vi "TTB Convert.vi"(0 "time of 1st frame, sec since 1/1/04":dbl format="%.2f", 2 "First element of TTB values":u32, 3 "Current element of TTB values":u32) -> (5 "TTB Cluster Out":cluster{i32, u16, i16, i16})   [LabVIEW 2011]
doc: "Time Table Conversion VI.\n\n This VI converts a single element of the time table array by subtracting the first element from the current element. The number found is how many milliseconds have passed since the first frame grab. This information is stored in the TTB cluster in two ways: First, the number of seconds since 1970 is saved in the first slot of the cluster, then the number of milliseconds (three decimal places recorded) is saved in the second slot. The remaining two slots of the cluster are filled with zeros, as they are useless placeholders to make our TTB compliant with the C++ version.\n The VI divides the # of millisecs since the first frame by 1000 to achieve two goals: First, the quotient is added to the # of seconds to get the true # of seconds since the first frame grab, and then the remainder is passed to the cluster, since it is the true # of milliseconds."
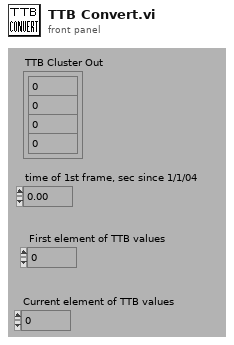
[diagram p1: front panel]
types:
  T1 = cluster{"second":i32, "minute":i32, "hour":i32, "day of month":i32, "month":i32, "year":i32, "day of week":i32, "day of year":i32, "is DST":i32}
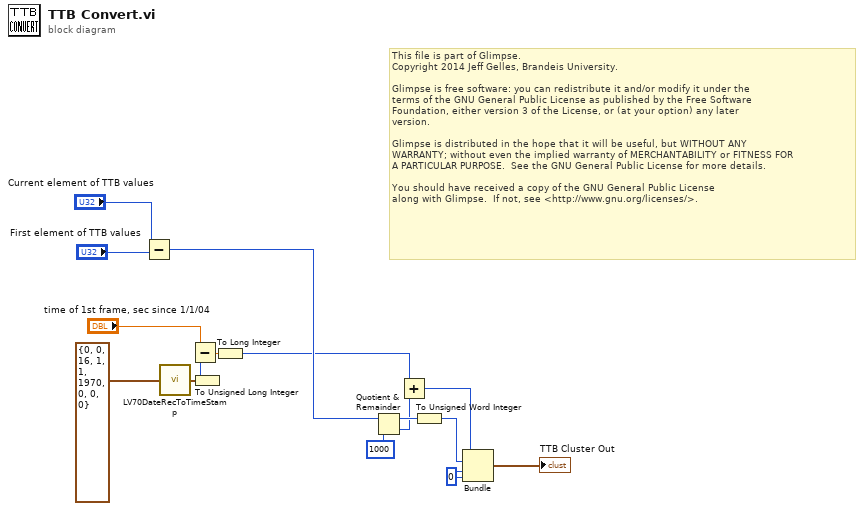
[diagram p0: block diagram]
diagram:
  w11 = i16 0
  # "This file is part of Glimpse. \nCopyright 2014 Jeff Gelles, Brandeis University.    \n\nGlimpse is free software: you can redistribute it and/or modify it under the \nterms of the GNU General Public License as published by the Free Software \nFoundation, either version 3 of the License, or (at your option) any later \nversion.\n\nGlimpse is distributed in the hope that it will be useful, but WITHOUT ANY \nWARRANTY; without even the implied warranty of MERCHANTABILITY or FITNESS FOR \nA PARTICULAR PURPOSE.  See the GNU General Public License for more details.\n\nYou should have received a copy of the GNU General Public License\nalong with Glimpse.  If not, see <http://www.gnu.org/licenses/>."
  n1 = Subtract(x="Current element of TTB values", y="First element of TTB values") -> (x-y=w6:u32)
  n2 = call <vilib>:"LV70DateRecToTimeStamp.vi"("date time rec"=T1 {"second"=0, "minute"=0, "hour"=16, "day of month"=1, "month"=1, "year"=1970, "day of week"=0, "day of year"=0, "is DST"=0}) -> ("Time Stamp"=w1:timestamp)
  n3 = To Unsigned Long Integer(number=w1) -> (unsigned 32bit integer=w15:u32)
  n4 = Subtract(x="time of 1st frame, sec since 1/1/04", y=w15) -> (x-y=w14:dbl)
  n5 = To Long Integer(number=w14) -> (32bit integer=w5:i32)
  n6 = Quotient & Remainder(x=w6, y=u32 1000) -> (x-y*floor(x/y)=w10:u32, floor(x/y)=w8:u32)
  n7 = Add(x=w5, y=w8) -> (x+y=w4:u32)
  n8 = To Unsigned Word Integer(number=w10) -> (unsigned 16bit integer=w9:u16)
  n9 = Bundle(w4, w9, w11, w11) -> (→"TTB Cluster Out":cluster{u32, u16, i16, i16})  [unwired: 1 out]
